vi "Data Write.vi"(7 "Retry Attempts (0)":i32 min=0, 8 "error in (no error)":errorcluster, 10 "Command":string, 11 "VISA Refnum in":refnum<visa-resource-name>) -> (0 "error out":errorcluster, 3 "VISA Refnum out":refnum<visa-resource-name>)   [LabVIEW 2018, in "Omega Platinum Series.lvlib"]
doc: "Performs a VISA Write to the given VISA port with the given command. The write action will be retried upon failure up to N times, where N is the Retry Attempts given, where N >= 0. Values less than zero will be treated as zero. The first wait time is 1 second, which doubles in subsequent retry wait times, similar to TCP communications prior to any segments being received.\n\nFor example, attempt 1 (0 retries) = 1 second wait; attempt 2 (1 retry) = 2 second wait; attempt 3 (2 retries) = 4 second wait. The number of seconds waited on a given retry attempt can be represented with the formula 2^n, where n is the number of retries attempted."
uses:
  <instrlib>/Omega Platinum Series/Omega Platinum Series.lvlib
  <vilib>/Utility/sysdir.llb/System Directory Type.ctl
panel:
  out "Retries":i32
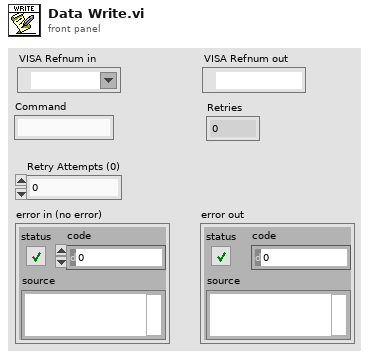
[diagram p1: front panel]
types:
  T1 = typedef "System Directory Type.ctl" = i32
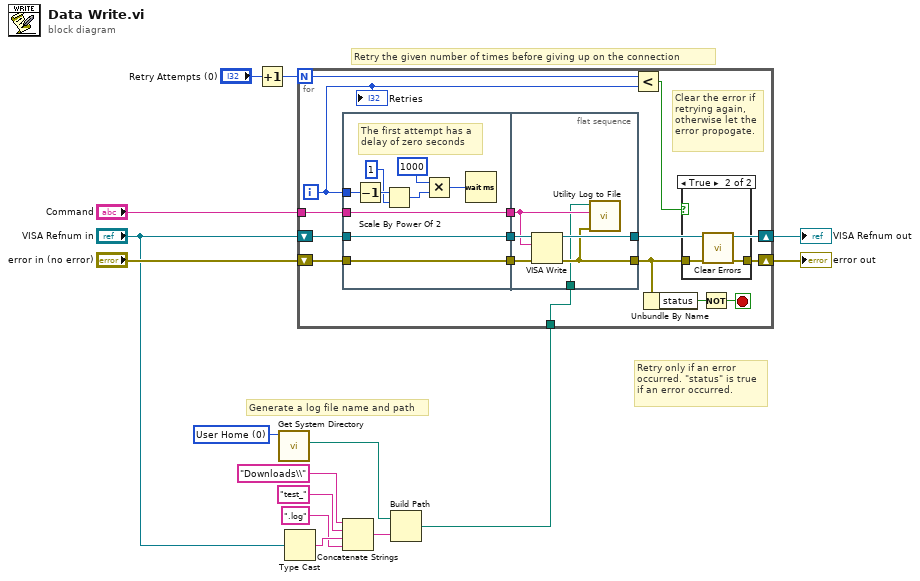
[diagram p0: block diagram]
diagram:
  w8 = T1 0 items=["User Home"=0, "User Desktop"=1, "User Documents"=2, "User Application Data"=3, "User Preferences"=4, "User Temporary"=5, "Public Documents"=6, "Public Application Data"=7, "Public Preferences"=8, "Public Cache"=13, "System Core Libraries"=9, "System Installed Libraries"=10, "Application Files"=11, "Boot Volume Root"=12] ("system directory type")
  # "Retry only if an error\noccurred. \"status\" is true\nif an error occurred."
  # "Retry the given number of times before giving up on the connection"
  # "Generate a log file name and path"
  n1 = Increment(x="Retry Attempts (0)") -> (x+1=w1:i32)
  n2 = call <vilib>:"Get System Directory.vi"("system directory type"=w8) -> ("system directory"=w4:path)  [unwired: 10 in]
  n3 = Type Cast(x="VISA Refnum in") -> (*(type *) &x=w10:string)  [unwired: 1 in]
  n4 = Concatenate Strings("Downloads\\", "test_", w10, ".log") -> (w5:string)
  n5 = Build Path(base path=w4, name or relative path=w5) -> (appended path=w3:path)
  n6 = for {
    N: w1 -> [w17]
    tunnel: "Command" -> [w27]
    tunnel: w3 -> [w23]
    shift-right: [w30] -> w15
    shift-left: "VISA Refnum in" -> [w29]
    shift-right: [w19] -> w12
    shift-left: "error in (no error)" -> [w28]
    i -> [w16]
    stop <- w20 stop-if-true
    # "Clear the error if\nretrying again,\notherwise let the\nerror propogate."
    n7 = flat-sequence {
      tunnel: w27 -> [w40]
      tunnel: w28 -> [w41]
      tunnel: w29 -> [w42]
      tunnel: [w42] -> w26
      tunnel: [w41] -> w25
      tunnel: [w40] -> w24
      tunnel: w16 -> [w39]
      tunnel: [w48] -> w30
      tunnel: [w45] -> w22
      tunnel: w23 -> [w43]
      tunnel: w26 -> [w47]
      tunnel: w25 -> [w46]
      tunnel: w24 -> [w44]
      frame #0 {
        # "The first attempt has a \ndelay of zero seconds"
        n8 = Decrement(x=w39) -> (x-1=w35:i32)
        n9 = Scale By Power Of 2(n=w35, x=1) -> (x*2^n=w38:i32)
        n10 = Multiply(x=1000, y=w38) -> (x*y=w36:i32)
        n11 = Wait (ms)(milliseconds to wait=w36) -> ()  [unwired: 1 out]
      }
      frame #1 {
        n12 = VISA Write(VISA resource name=w47, write buffer=w44, error in (no error)=w46) -> (VISA resource name out=w48:refnum<visa-resource-name>, error out=w45:errorcluster)  [unwired: 1 out]
        n13 = call <instrlib>:"Utility Log to File.vi"("error in (no error)"=w45, "Command"=w44, "Log File Path"=w43) -> ()  [unwired: 8 in, 1 out]
      }
    }
    n14 = Less?(x=w17, y=w16) -> (x < y?=w18:bool)
    n15 = Unbundle By Name(w22) -> ("status"=w21:bool)
    n16 = case shown="True" w18 {
      tunnel: w22 -> [w31 w33]
      tunnel: [w31 w32] -> w19
      frame False {
      }
      frame True {
        n17 = call <vilib>:"Clear Errors.vi"("error in (no error)"=w33) -> ("error out"=w32:errorcluster)  [unwired: 5 in, 1 out]
      }
    }
    n18 = Not(x=w21) -> (.not. x?=w20:bool)
    "Retries" <- w16
  }
  "VISA Refnum out" <- w15
  "error out" <- w12
